vi "Download to Device.vi"(6 "Verified":bool=TRUE, 8 "error in (no error)":errorcluster, 9 "Specified Address?":bool, 10 "Memory Address":u32=134217728 format="%08x", 11 "FW Path":path) -> (0 "error out":errorcluster, 3 "Download OK?":bool)   [LabVIEW 2015, in "ST-Link.lvlib"]
doc: "下载固件到芯片。\nFW Path: 指定固件文件路径，支持三种格式（.bin / .hex / .srec）；\nMemory Address: 指定烧录的起始内存地址，STM32的Flash映射地址是从0x08000000开始的；\nSpecified Address?: 是否按照指定的地址开始下载；\nVerified: 是否启用验证功能，使能后会在下载完进行校验，默认是使能的；\n\n[Download OK?]: 返回下载状态；"
uses:
  ST-Link.lvlib
panel:
  out "standard output":string
  # "(support .hex/.bin/.srec)"
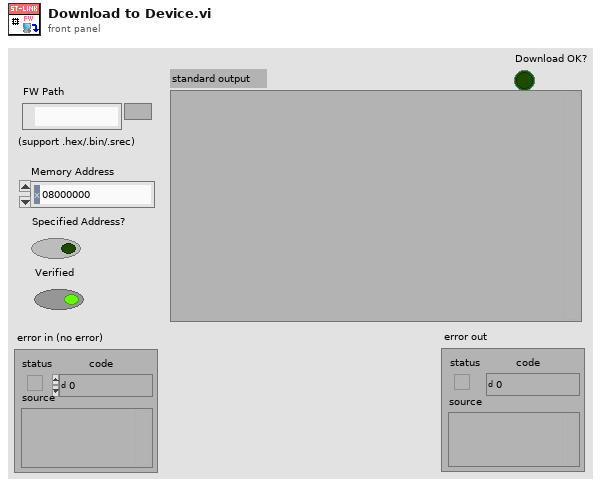
[diagram p1: front panel]
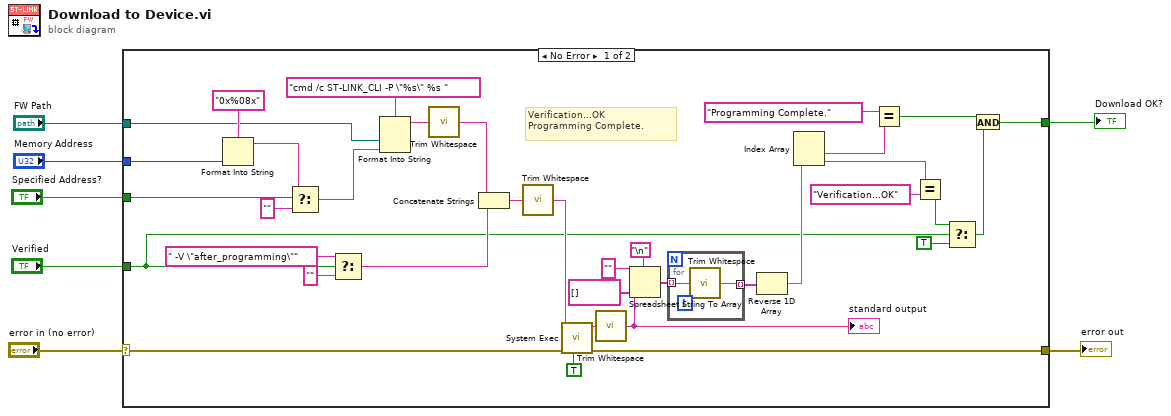
[diagram p0: block diagram]
diagram:
  n1 = case shown="No Error" "error in (no error)" {
    selector: "error in (no error)" -> [w42 w46]
    tunnel: [w41 w46] -> w6
    tunnel: "Specified Address?" -> [w40 _]
    tunnel: "Memory Address" -> [w38 _]
    tunnel: "FW Path" -> [w34 _]
    tunnel: "Verified" -> [w13 _]
    tunnel: [w9 _] -> w1
    frame No Error {
      # "Verification...OK\nProgramming Complete."
      n2 = Format Into String(format string="0x%08x", w38) -> (resulting string=w37:string)  [unwired: 2 in, 1 out]
      n3 = Select(t=w37, s=w40, f="") -> (s? t:f=w33:string)
      n4 = Select(t=" -V \"after_programming\"", s=w13, f="") -> (s? t:f=w28:string)
      n5 = Format Into String(format string="cmd /c ST-LINK_CLI -P \"%s\" %s " ("command line"), w34, w33) -> (resulting string=w32:string)  [unwired: 2 in, 1 out]
      n6 = call <vilib>:"Trim Whitespace.vi"("string"=w32) -> ("trimmed string"=w29:string)  [unwired: 1 in]
      n7 = Concatenate Strings(w29, w28) -> (w27:string)
      n8 = call <vilib>:"Trim Whitespace.vi"("string"=w27) -> ("trimmed string"=w26:string)  [unwired: 1 in]
      n9 = call <vilib>:"System Exec.vi"("run minimized? (F)"=TRUE, "error in (no error)"=w42, "command line"=w26) -> ("error out"=w41:errorcluster, "standard output"=w25:string)  [unwired: 5 in, 2 out]
      n10 = call <vilib>:"Trim Whitespace.vi"("string"=w25) -> ("trimmed string"=w8:string)  [unwired: 1 in]
      "standard output" <- w8
      n11 = Spreadsheet String To Array(delimiter (Tab)="\n", format string="", spreadsheet string=w8, array type (2D Dbl)=string[] []) -> (array=w21:string[])
      n12 = for {
        tunnel: w21 -> [w45] mode=indexing
        tunnel: [w44] -> w20 mode=indexing
        n13 = call <vilib>:"Trim Whitespace.vi"("string"=w45) -> ("trimmed string"=w44:string)  [unwired: 1 in]
      }
      n14 = Reverse 1D Array(array=w20) -> (reversed array=w19:string[])
      n15 = Index Array(array=w19) -> (element #1=w18:string, element #2=w17:string)  [unwired: 2 in]
      n16 = Equal?(x="Programming Complete." ("y"), y=w18) -> (x = y?=w14:bool)
      n17 = Equal?(x=w17, y="Verification...OK") -> (x = y?=w12:bool)
      n18 = Select(t=w12, s=w13, f=TRUE) -> (s? t:f=w10:bool)
      n19 = And(x=w14, y=w10) -> (x .and. y?=w9:bool)
    }
    frame Error {
    }
  }
  "error out" <- w6
  "Download OK?" <- w1
